vi "Add.vi"() -> ()   [LabVIEW 2018]
panel:
  out "error out":errorcluster
  in  "B":i32=6
  in  "A":i32=5
  out "C":i32
  # "+"
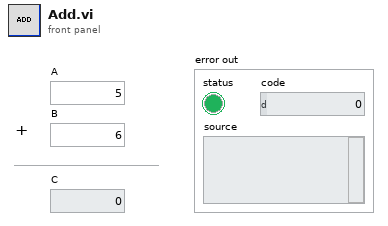
[diagram p1: front panel]
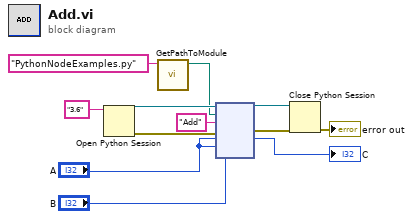
[diagram p0: block diagram]
diagram:
  n1 = Open Python Session(python version="3.6" ("Python version")) -> (session out=w12:refnum<k35>, error out=w5:errorcluster)  [unwired: 2 in]
  n2 = call "GetPathToModule.vi"("module name"="PythonNodeExamples.py") -> ("path to module"=w1:path)  [unwired: 10 in]
  n3 = node(w12, w1, "Add" ("function name"), w5, "A", "A", "B") -> (w11:refnum<k35>, w4:errorcluster, →"C":i32)  [unwired: 2 in, 2 out]
  n4 = Close Python Session(session in=w11, error in=w4) -> (11:→"error out":errorcluster)
